vi "Get Basic Audio File Info.vi"(8 "error in (no error)":errorcluster, 11 "Audio File Refnum In":T1) -> (0 "error out":errorcluster, 1 "sample_rate":u32, 2 "channels":u32, 3 "Audio File Refnum Out":T1)   [LabVIEW 2020, in "G-Audio.lvlib"]
doc: "Get basic audio information about the file."
uses:
  G-Audio.lvlib
  Controls/Audio File Refnum.ctl
  <vilib>/Utility/error.llb/Error Cluster From Error Code.vi
  lib/g_audio_32.dll
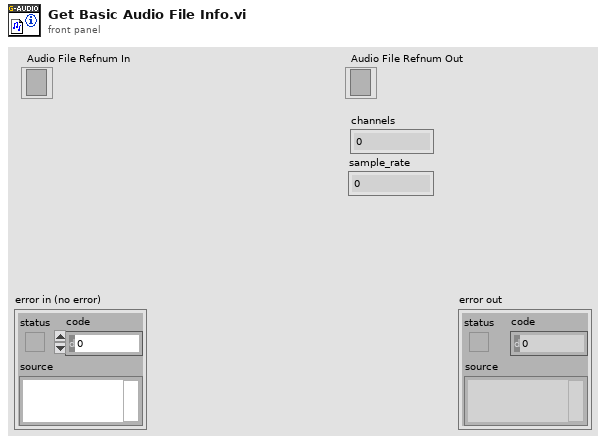
[diagram p1: front panel]
types:
  T1 = typedef "G-Audio.lvlib/Audio File Refnum.ctl" = refnum<file>
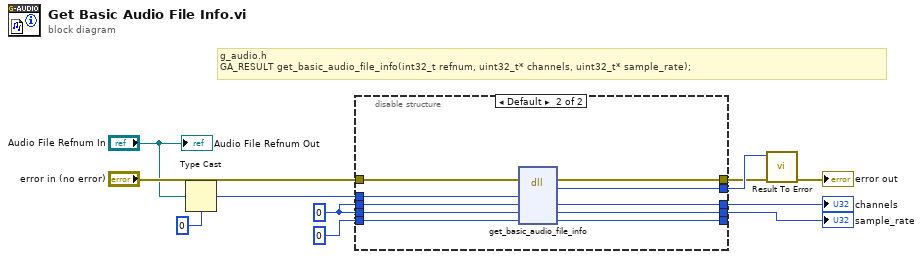
[diagram p0: block diagram]
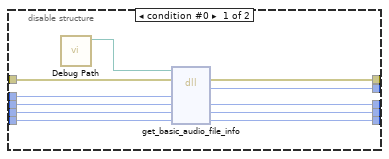
[diagram p2: hidden frame]
diagram:
  w7 = u32 0
  # "g_audio.h\nGA_RESULT get_basic_audio_file_info(int32_t refnum, uint32_t* channels, uint32_t* sample_rate);"
  n1 = Type Cast(type=0, x="Audio File Refnum In") -> (*(type *) &x=w8:i32)
  n2 = disable-structure shown="Default" {
    disable-tunnel: "error in (no error)" -> [w22 w32]
    disable-tunnel: [w15 w25] -> w4
    disable-tunnel: [w21 w31] -> w3
    disable-tunnel: [w16 w26] -> w5
    disable-tunnel: w8 -> [w20 w30]
    disable-tunnel: w7 -> [w19 w29]
    disable-tunnel: w7 -> [w18 w28]
    disable-tunnel: [w17 w27] -> w6
    disable-tunnel: u64 0 -> [w13 w24]
    disable-tunnel: [w12 w23] -> _
    frame condition #0 {
      n3 = call "Debug Path.vi"() -> ("Debug Path"=w14:path)  [unwired: 11 in]
      n4 = dll-call lib="?" fn="get_basic_audio_file_info"(path in=w14, error in=w22, "refnum"=w20, "channels"=w19, "sample_rate"=w18, "read_offset"=w13) -> (error out=w21:errorcluster, "result"=w15:i32, "channels"=w17:u32, "sample_rate"=w16:u32, "read_offset"=w12:u64)  [unwired: 2 in, 1 out]
    }
    frame condition #1 (active) {
      n5 = dll-call lib="C:/github/dataflowg/g-audio/src/LabVIEW/G-Audio/lib/g_audio_*.*" fn="get_basic_audio_file_info"(error in=w32, "refnum"=w30, "channels"=w29, "sample_rate"=w28, "read_offset"=w24) -> (error out=w31:errorcluster, "result"=w25:i32, "channels"=w27:u32, "sample_rate"=w26:u32, "read_offset"=w23:u64)  [unwired: 3 in, 1 out]
    }
  }
  "channels" <- w6
  "sample_rate" <- w5
  n6 = call "Result To Error.vi"("error in (no error)"=w3, "Result Code"=w4) -> ("error out"=→"error out":errorcluster)  [unwired: 9 in]
  "Audio File Refnum Out" <- "Audio File Refnum In"
